vi "FTW-Package-Request-Reply.vi"(8 "FTW: Reply Error":errorcluster caption="error in", 11 "FTW Incoming Request":refnum<class "FTW-Package-IncomingRequest.lvclass">) -> (0 "error out":errorcluster, 2 "Timed out?":bool)   [LabVIEW 2013, in "FTW-Package-IncomingRequest.lvclass"]
uses:
  FTW-Package-IncomingRequest.lvclass
  FTW-Package-IncomingRequest.lvclass/FTW-Package-IncomingRequest.ctl
  Endpoint/FTW-Endpoint.lvclass
panel:
  # "Inputs"
  # "Outputs"
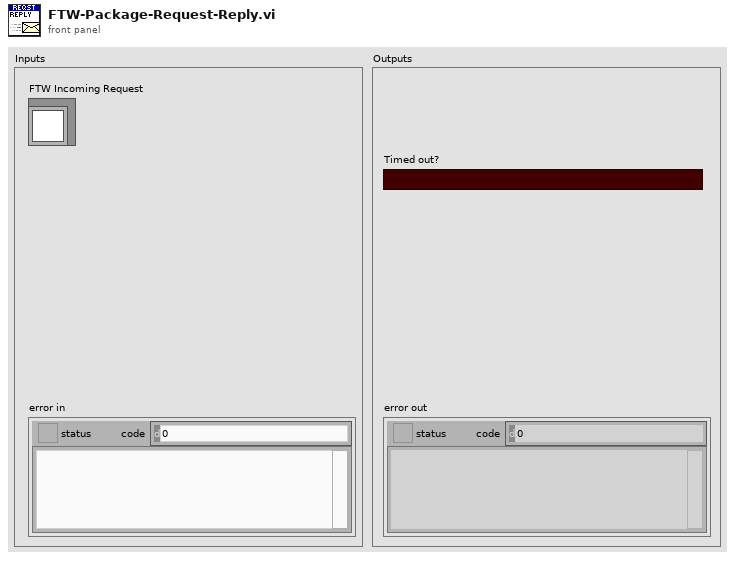
[diagram p1: front panel]
types:
  T1 = typedef "FTW-Message.ctl" = cluster{"Header":string, "Body":string, "Metadata":string}
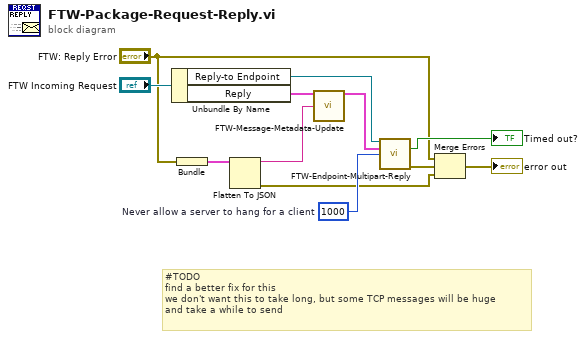
[diagram p0: block diagram]
diagram:
  w9 = 1000  # Never allow a server to hang for a client
  # "#TODO\nfind a better fix for this\nwe don't want this to take long, but some TCP messages will be huge\nand take a while to send"
  n1 = Unbundle By Name("FTW Incoming Request") -> ("Reply-to Endpoint"=w11:refnum<class "FTW-Endpoint.lvclass">, "Reply"=w3:T1)
  n2 = Bundle("FTW: Reply Error"="FTW: Reply Error") -> (w4:cluster{"FTW: Reply Error":errorcluster})  [unwired: 1 in]
  n3 = Flatten To JSON(anything=w4) -> (JSON string=w1:string, 11:w6:errorcluster)  [unwired: 2 in]
  n4 = call "FTW-Message-Metadata-Update.vi"("Message In"=w3, "Metadata"=w1) -> ("Message"=w2:T1)  [unwired: 12 in, 1 out]
  n5 = call-dynamic "FTW-Endpoint-Multipart-Reply.vi"("FTW Endpoint"=w11, "Message"=w2, "Timeout"=w9) -> ("Timed out?"=→"Timed out?":bool, "error out"=w10:errorcluster)  [unwired: 10 in, 1 out]
  n6 = Merge Errors("FTW: Reply Error", w10, w6) -> (→"error out":errorcluster)
